vi "Set_Tunnel_Speed_Multi.vi"(3 "Simulate/Run":T3, 5 "Traverse line":T4 {"Row Duration (mins)" format="%#.1f"; "Row No" min=0; "Trace Gas Concentration (%)" min=0.0 format="%#.2f"; "Emission Rate (l/min)" format="%#.2f"; "Tunnel Speed" format="%#.2f"; "Start X" format="%#.2f"; "Start Y" format="%#.2f"; "Start Z" format="%#.2f"; "End X" format="%#.2f"; "End Y" format="%#.2f"; "End Z" format="%#.2f"; "Averaging time (min)" min=0.0 format="%#.1f"}) -> (0 "Status Cluster":T1)   [LabVIEW 2010]
uses:
  Traverse_cluster.ctl
  Spacing.ctl
  Controls/Multi_run_mode.ctl
  Controls/User_Specific_mode.ctl
  Status_Cluster.ctl
  Multi_Run_Status.ctl
  ADAM Client/Sub VIs/ADAM Controls/Tunnel_speed_mode.ctl
  Globals/Preference_global.vi
panel:
  # "X           Y            Z"
  # "Start"
  # "End"
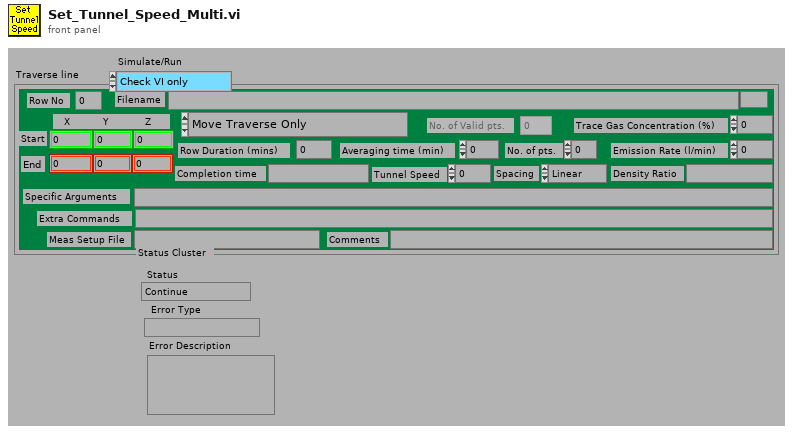
[diagram p1: front panel]
types:
  T1 = typedef "Status_Cluster.ctl" = cluster{"Status":T2, "Error Type":string, "Error Description":string}
  T2 = typedef "Multi_Run_Status.ctl" = enum16{"Continue", "Jump to Next Point", "Jump to Next Row", "Jump To Fall Back", "Terminate Run"}
  T3 = typedef "User_Specific_mode.ctl" = enum16{"Check VI only", "Run VI"}
  T4 = typedef "Traverse_cluster.ctl" = cluster{"Start X":dbl, "Start Y":dbl, "Start Z":dbl, "End X":dbl, "End Y":dbl, "End Z":dbl, "No. of pts.":i32, "Spacing":T5, "Filename":path, "Tunnel Speed":dbl, "Averaging time (min)":dbl, "Extra Commands":string, "Specific Arguments":string, "Emission Rate (l/min)":dbl, "Trace Gas Concentration (%)":dbl, "Density Ratio":string, "Comments":string, "Row No":i32, "Row Type Selector":T6, "Completion time":string, "Row Duration (mins)":dbl, "No. of Valid pts.":i32, "Meas Setup File":string}
  T5 = typedef "Spacing.ctl" = enum16{"Linear", "Log", "Gauss", "Specified", "N/A"}
  T6 = typedef "Multi_run_mode.ctl" = enum16{"Move Traverse Only", "Set Tunnel Speed Only", "Set Source Only", "Set Measurement Conditions", "Single Measurement", "Vertical Profile", "Lateral Profile", "Longitudinal Profile", "Explore Volume", "Multi-Axis Profile", "Auto Calibrate", "Meas Fast FID Bkgnd", "Check Beam Power", "Scanning Valve Measurement", "Run VI Named:", "Set ADAM Ch", "Wait (minutes)", "Send Message", "Synchronize With:", "Fall Back to this Row", "Turn Off Row Repeating", "Blank Row"}
  T7 = typedef "Tunnel_speed_mode.ctl" = enum16{"Set Speed", "Set Speed then wait", "Is tunnel speed allowable?"}
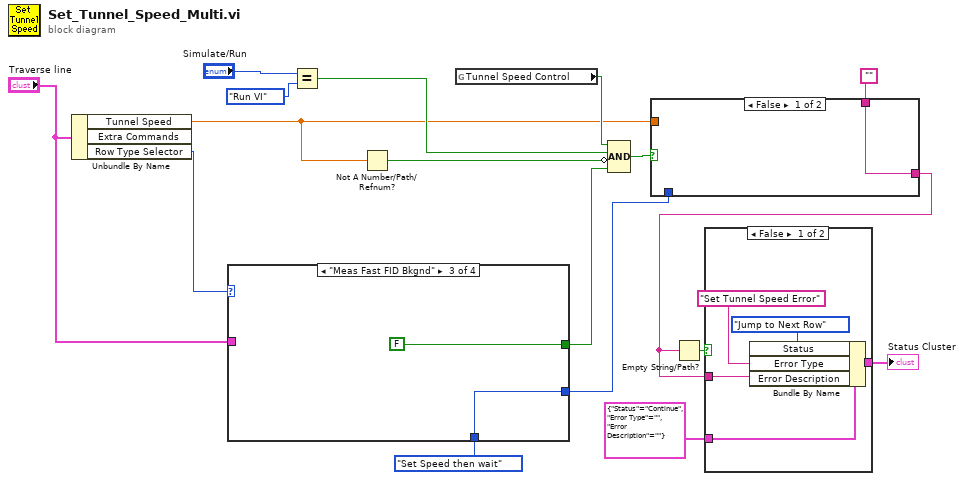
[diagram p0: block diagram]
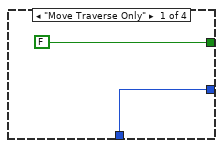
[diagram p3: hidden frame]
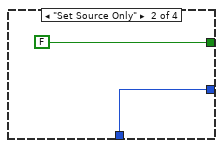
[diagram p4: hidden frame]
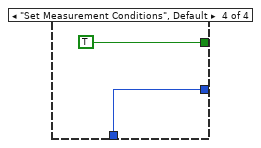
[diagram p5: hidden frame]
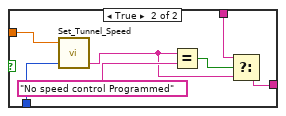
[diagram p6: hidden frame]
diagram:
  n1 = Unbundle By Name("Traverse line") -> ("Tunnel Speed"=w2:dbl, "Row Type Selector"=w13:T6)  [unwired: 1 out]
  n2 = case shown="\"Meas Fast FID Bkgnd\"" w13 {
    tunnel: [FALSE FALSE FALSE TRUE] -> w5
    tunnel: "Traverse line" -> [_ _ _ _]
    tunnel: [w18 w20 w22 w24] -> w11
    tunnel: Tunnel_speed_mode."Set Speed then wait" ("Mode") -> [w18 w20 w22 w24]
    frame "Move Traverse Only" {
    }
    frame "Set Source Only" {
    }
    frame "Meas Fast FID Bkgnd" {
    }
    frame "Set Measurement Conditions", Default {
    }
  }
  n3 = Equal?(x="Simulate/Run", y=User_Specific_mode."Run VI" ("Simulate/Run")) -> (x = y?=w15:bool)
  n4 = Not A Number/Path/Refnum?(number/path/refnum=w2) -> (NaN/Path/Refnum?=w1:bool)
  n5 = global read "Preference_global.vi" "Tunnel Speed Control"() -> (w3:bool)
  n6 = Compound Arithmetic op=AND(w3, w15, invert w1, w5) -> (w16:bool)
  n7 = case shown="False" w16 {
    tunnel: w2 -> [_ w27]
    tunnel: w11 -> [_ w33]
    tunnel: [w26 w28] -> w6
    tunnel: "" -> [w26 w30]
    frame False {
    }
    frame True {
      n8 = call "Set_Tunnel_Speed.vi"("Mode"=w33, "Tunnel Velocity m/s"=w27) -> ("Error String"=w29:string)  [unwired: 1 in, 2 out]
      n9 = Equal?(x=w29, y="No speed control Programmed" ("Error String")) -> (x = y?=w31:bool)
      n10 = Select(t=w30, s=w31, f=w29) -> (s? t:f=w28:string)
    }
  }
  n11 = Empty String/Path?(string/path=w6) -> (empty?=w8:bool)
  n12 = case shown="False" w8 {
    tunnel: T1 {"Status"=enum."Continue", "Error Type"="", "Error Description"=""} ("Status Cluster") -> [w38 w39]
    tunnel: [w37 w39] -> w7
    tunnel: w6 -> [w34 _]
    frame False {
      n13 = Bundle By Name(cluster=w38, "Status"=Multi_Run_Status."Jump to Next Row", "Error Type"="Set Tunnel Speed Error" ("Bundle Element"), "Error Description"=w34) -> (w37:T1)
    }
    frame True {
    }
  }
  "Status Cluster" <- w7
